vi "strings to line.vi"(11 "strings":string[](array[string])) -> (3 "line":T1)   [LabVIEW 2013, in "Modbus Slave editor node.lvclass"]
doc: "Platypus Framework 1.0.1.65\nNI Systems Engineering - National Instruments"
uses:
  Modbus Slave editor node.lvclass
  <vilib>/NI/Tag Bus/tag/Data Type.ctl
  <vilib>/NI/Tag Bus/tag/tag descriptor.lvclass
  table line.ctl
  permissions.ctl
  module/module channel/Modbus Module Channel.lvclass
  module/module channel/data bank type.ctl
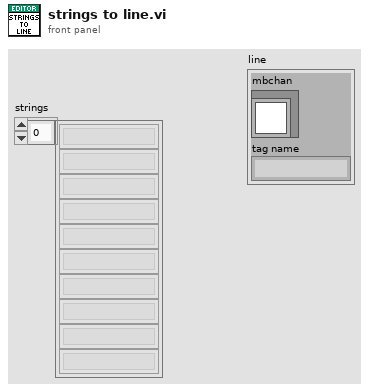
[diagram p1: front panel]
types:
  T1 = typedef "Modbus Slave editor node.lvclass/table line.ctl" = cluster{"mbchan":refnum<class "Modbus Module Channel.lvclass">, "tag name":string}
  T2 = typedef "Modbus Module Channel.lvclass/data bank type.ctl" = enum16{"coils", "discrete inputs", "input registers", "holding registers"}
  T3 = typedef "Modbus Slave editor node.lvclass/permissions.ctl" = enum32{"Read from MB", "Write to MB"}
  T4 = typedef "tag bus.lvlib/tag descriptor.lvclass/Data Type.ctl" = enum16{"Double", "Single", "I64", "I32", "I16", "I8", "U64", "U32", "U16", "U8", "Boolean", "String", "Array of Double", "Array of Single", "Array of I64", "Array of I32", "Array of I16", "Array of I8", "Array of U64", "Array of U32", "Array of U16", "Array of U8", "Array of Boolean", "Array of String"}
  T5 = typedef "TBM channel.lvclass/channel classification.ctl" = enum16{"input data", "output data", "processing parameter", "processing result"}
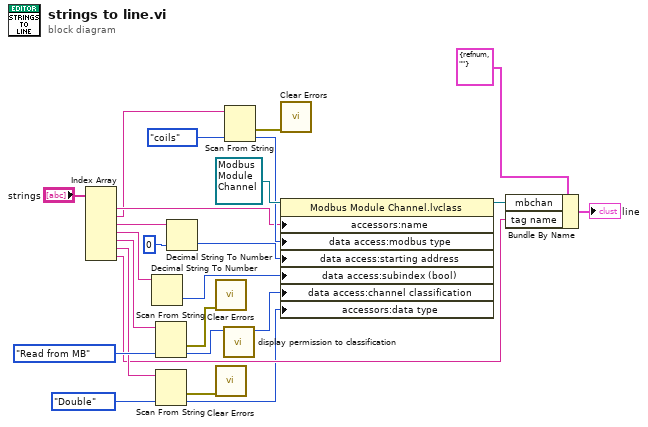
[diagram p0: block diagram]
diagram:
  n1 = Index Array(array="strings") -> (element #1=w2:string, element #2=w1:string, element #3=w10:string, element #4=w9:string, element #5=w18:string, element #6=w16:string, element #7=w15:string)  [unwired: 7 in]
  n2 = Decimal String To Number(string=w9) -> (number=w8:i32)  [unwired: 2 in, 1 out]
  n3 = Scan From String(input string=w18, default 1=permissions."Read from MB" ("direction")) -> (error out=w20:errorcluster, output 1=w17:T3)  [unwired: 3 in, 2 out]
  n4 = Scan From String(input string=w16, default 1=Data_Type."Double" ("data type")) -> (error out=w22:errorcluster, output 1=w12:T4)  [unwired: 3 in, 2 out]
  n5 = Decimal String To Number(string=w10, default (0L)=u16 0 ("default (0 I32)")) -> (number=w7:u16)  [unwired: 1 in, 1 out]
  n6 = call <vilib>:"Clear Errors.vi"("error in (no error)"=w20) -> ()  [unwired: 6 in, 1 out]
  n7 = call <vilib>:"Clear Errors.vi"("error in (no error)"=w22) -> ()  [unwired: 6 in, 1 out]
  n8 = call "display permission to classification.vi"("display permissions"=w17) -> ("channel classification"=w11:T5)  [unwired: 10 in]
  n9 = Scan From String(input string=w1, default 1=data_bank_type."coils" ("modbus type")) -> (error out=w5:errorcluster, output 1=w3:T2)  [unwired: 3 in, 2 out]
  n10 = call <vilib>:"Clear Errors.vi"("error in (no error)"=w5) -> ()  [unwired: 6 in, 1 out]
  n11 = property class="Modbus Module Channel.lvclass"(reference=refnum<class "Modbus Module Channel.lvclass"> refnum ("Modbus Module Channel"), "accessors:name"=w2, "data access:modbus type"=w3, "data access:starting address"=w7, "data access:subindex (bool)"=w8, "data access:channel classification"=w11, "accessors:data type"=w12) -> (reference out=w13:refnum<class "Modbus Module Channel.lvclass">)  [unwired: 1 in, 1 out]
  n12 = Bundle By Name(cluster=T1 {"mbchan"=refnum, "tag name"=""} ("line"), "mbchan"=w13, "tag name"=w15) -> (→"line":T1)
